vi "Update.vi"(8 "error in (no error)":errorcluster, 10 "Message in":refnum<class "UpdateMessage.lvclass">, 11 "MeritFactor in":refnum<class "MeritFactor.lvclass">) -> (0 "error out":errorcluster, 3 "MeritFactor out":refnum<class "MeritFactor.lvclass">)   [LabVIEW 2012, in "MeritFactor.lvclass"]
doc: "The update method processes the command 'update'. \n\nThe command 'update' is used for receiving new values to be set to the private data of the class. This could be seen as a public set method for setting new parameters to the private class data."
uses:
  MeritFactor.lvclass
  <vilib>/Distrio/Murmex/UpdateMessage/UpdateMessage.lvclass
  MeritFactor.lvclass/MeritFactor.ctl
  <vilib>/Distrio/Murmex/Murmex/Murmex.lvclass
panel:
  # "This method is called when the UPDATE\ntrigger is sent. \n\nOverride this method when your component needs to\nrespond to this trigger. \n\nCall parent for proper implementation"
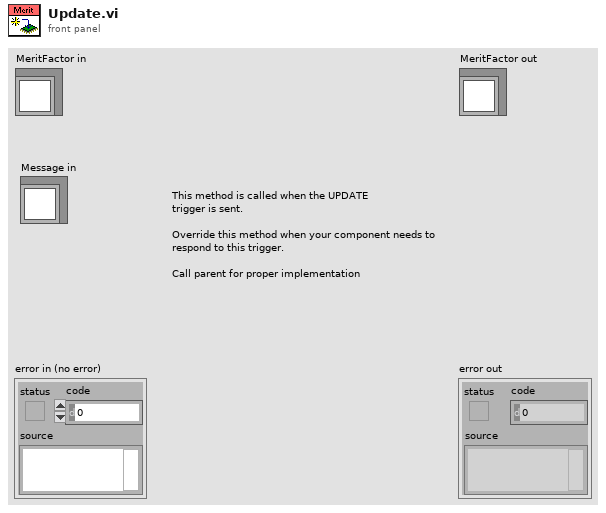
[diagram p1: front panel]
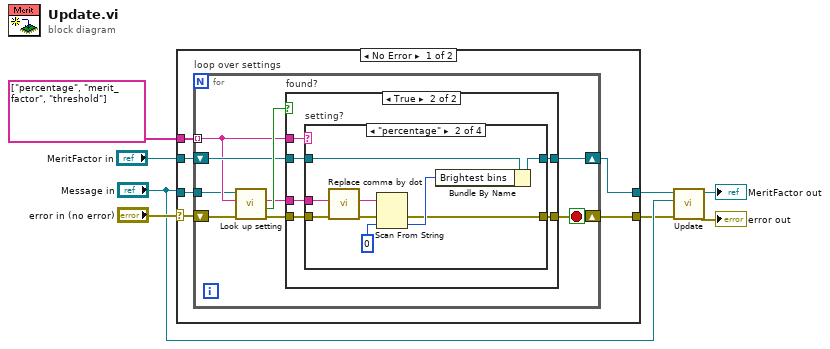
[diagram p0: block diagram]
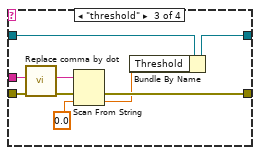
[diagram p4: hidden frame]
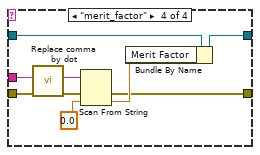
[diagram p5: hidden frame]
diagram:
  n1 = case shown="No Error" "error in (no error)" {
    selector: "error in (no error)" -> [w14 w58]
    tunnel: "MeritFactor in" -> [w13 w59]
    tunnel: string[] ["percentage", "merit_factor", "threshold"] -> [w12 _]
    tunnel: "Message in" -> [w11 _]
    tunnel: [w10 w58] -> w2
    tunnel: [w9 w59] -> w1
    frame No Error {
      n2 = for "loop over settings" {
        shift-right: [w15] -> w10
        shift-left: w14 -> [w23]
        shift-right: [w16] -> w9
        shift-left: w13 -> [w19]
        tunnel: w12 -> [w18] mode=indexing
        tunnel: w11 -> [w17]
        stop <- w15 stop-if-true
        n3 = call <vilib>:"Look up setting.vi"("error in (no error)"=w23, "tag name"=w18, "UpdateMessage in"=w17) -> ("error out"=w21:errorcluster, "found?"=w22:bool, "value"=w20:string)  [unwired: 5 in, 1 out]
        n4 = case "found?" shown="True" w22 {
          tunnel: w21 -> [w24 w31]
          tunnel: w20 -> [_ w30]
          tunnel: w19 -> [w25 w29]
          tunnel: w18 -> [_ w28]
          tunnel: [w25 w27] -> w16
          tunnel: [w24 w26] -> w15
          frame False {
          }
          frame True {
            n5 = case "setting?" shown="\"percentage\"" w28 {
              tunnel: w31 -> [w32 w39 w47 w55]
              tunnel: w30 -> [_ w40 w45 w56]
              tunnel: w29 -> [w33 w41 w44 w57]
              tunnel: [w33 w36 w42 w52] -> w27
              tunnel: [w32 w35 w46 w51] -> w26
              frame Default {
              }
              frame "percentage" {
                n6 = call <vilib>:"Replace comma by dot.vi"("input string"=w40) -> ("result string"=w34:string)  [unwired: 10 in]
                n7 = Scan From String(input string=w34, error in=w39, default 1=0 ("settings cluster.Brightest percentage")) -> (error out=w35:errorcluster, output 1=w37:i32)  [unwired: 2 in, 2 out]
                n8 = Bundle By Name(cluster=w41, "Brightest bins"=w37) -> (w36:refnum<class "MeritFactor.lvclass">)
              }
              frame "threshold" {
                n9 = call <vilib>:"Replace comma by dot.vi"("input string"=w45) -> ("result string"=w48:string)  [unwired: 10 in]
                n10 = Scan From String(input string=w48, error in=w47, default 1=sgl 0.0 ("settings cluster.Brightest percentage")) -> (error out=w46:errorcluster, output 1=w43:sgl)  [unwired: 2 in, 2 out]
                n11 = Bundle By Name(cluster=w44, "Threshold"=w43) -> (w42:refnum<class "MeritFactor.lvclass">)
              }
              frame "merit_factor" {
                n12 = call <vilib>:"Replace comma by dot.vi"("input string"=w56) -> ("result string"=w50:string)  [unwired: 10 in]
                n13 = Scan From String(input string=w50, error in=w55, default 1=0.0 ("settings cluster.Brightest percentage")) -> (error out=w51:errorcluster, output 1=w53:dbl)  [unwired: 2 in, 2 out]
                n14 = Bundle By Name(cluster=w57, "Merit Factor"=w53) -> (w52:refnum<class "MeritFactor.lvclass">)
              }
            }
          }
        }
      }
    }
    frame Error {
    }
  }
  n15 = call-parent "Update.vi"("error in (no error)"=w2, "Message in"="Message in", "Murmex in"=w1) -> ("error out"=→"error out":errorcluster, "Murmex out"=→"MeritFactor out":refnum<class "MeritFactor.lvclass">)  [unwired: 7 in]
